vi "Data Receiver_mod.vi"() -> ()   [LabVIEW 2024]
doc: "Demonstrates how to open a connection to a specified host and port, read the data being sent to the port, and display the data on a chart. This VI is designed to stop if the TCP connection is terminated.\n\n<B>Note:</B> Requires the Simple Data Server.vi located in the same library as this VI."
uses:
  <vilib>/Utility/TDMS File Viewer/NI_TDMS File Viewer.lvlib
panel:
  out "Time":string
  out "Bytes to read (dec)":i32
  out "Bytes to read (hex)":string
  out "Complete String after 'Bytes to read'":string
  out "Peak Powers":string[][](array[string])
  out "Peak Wavelengths":string[][](array[string])
  out "System Status":string[][](array[string])
  out "Qty of FBG's":string[](array[string])
  out "OpticalLineNumber":string[](array[string])
  out "Date":string
  out "LineNumber":string
  out "Qty of Optical Lines":string
  in  "Start":bool
  in  "stop":bool
  in  "Address":string="127.0.0.1"
  in  "Port":u16=2055 min=1025 step=1
  # "Instructions:\n1. Adjust the IP address and Port.\n2. Press START."
  # "Separated data"
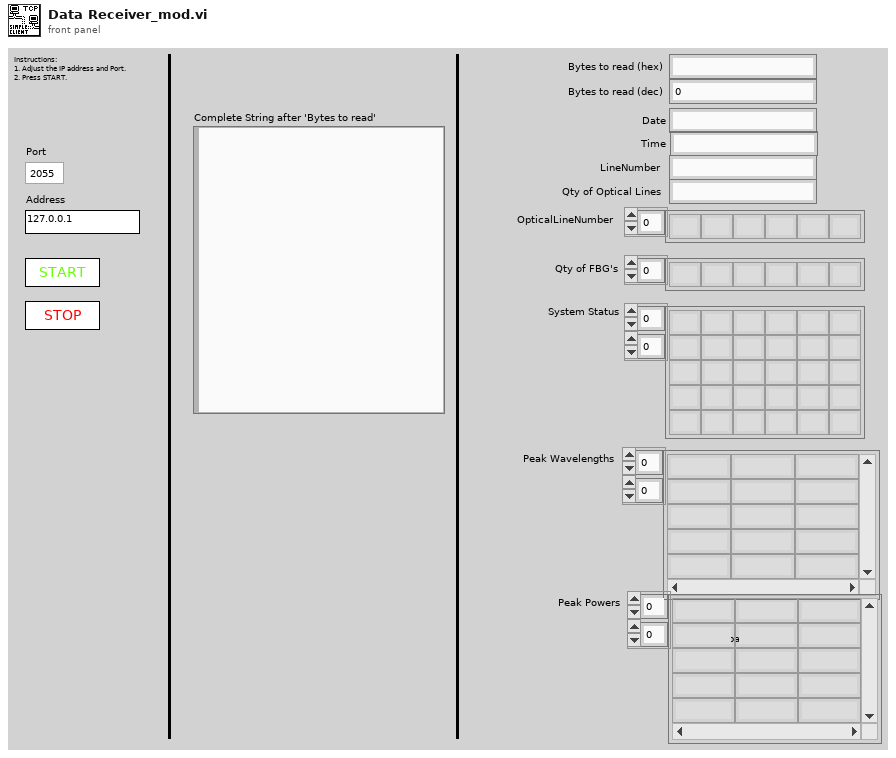
[diagram p1: front panel]
types:
  T1 = enum16{"open", "replace", "create", "open or create", "replace or create", "replace or create with confirmation"}
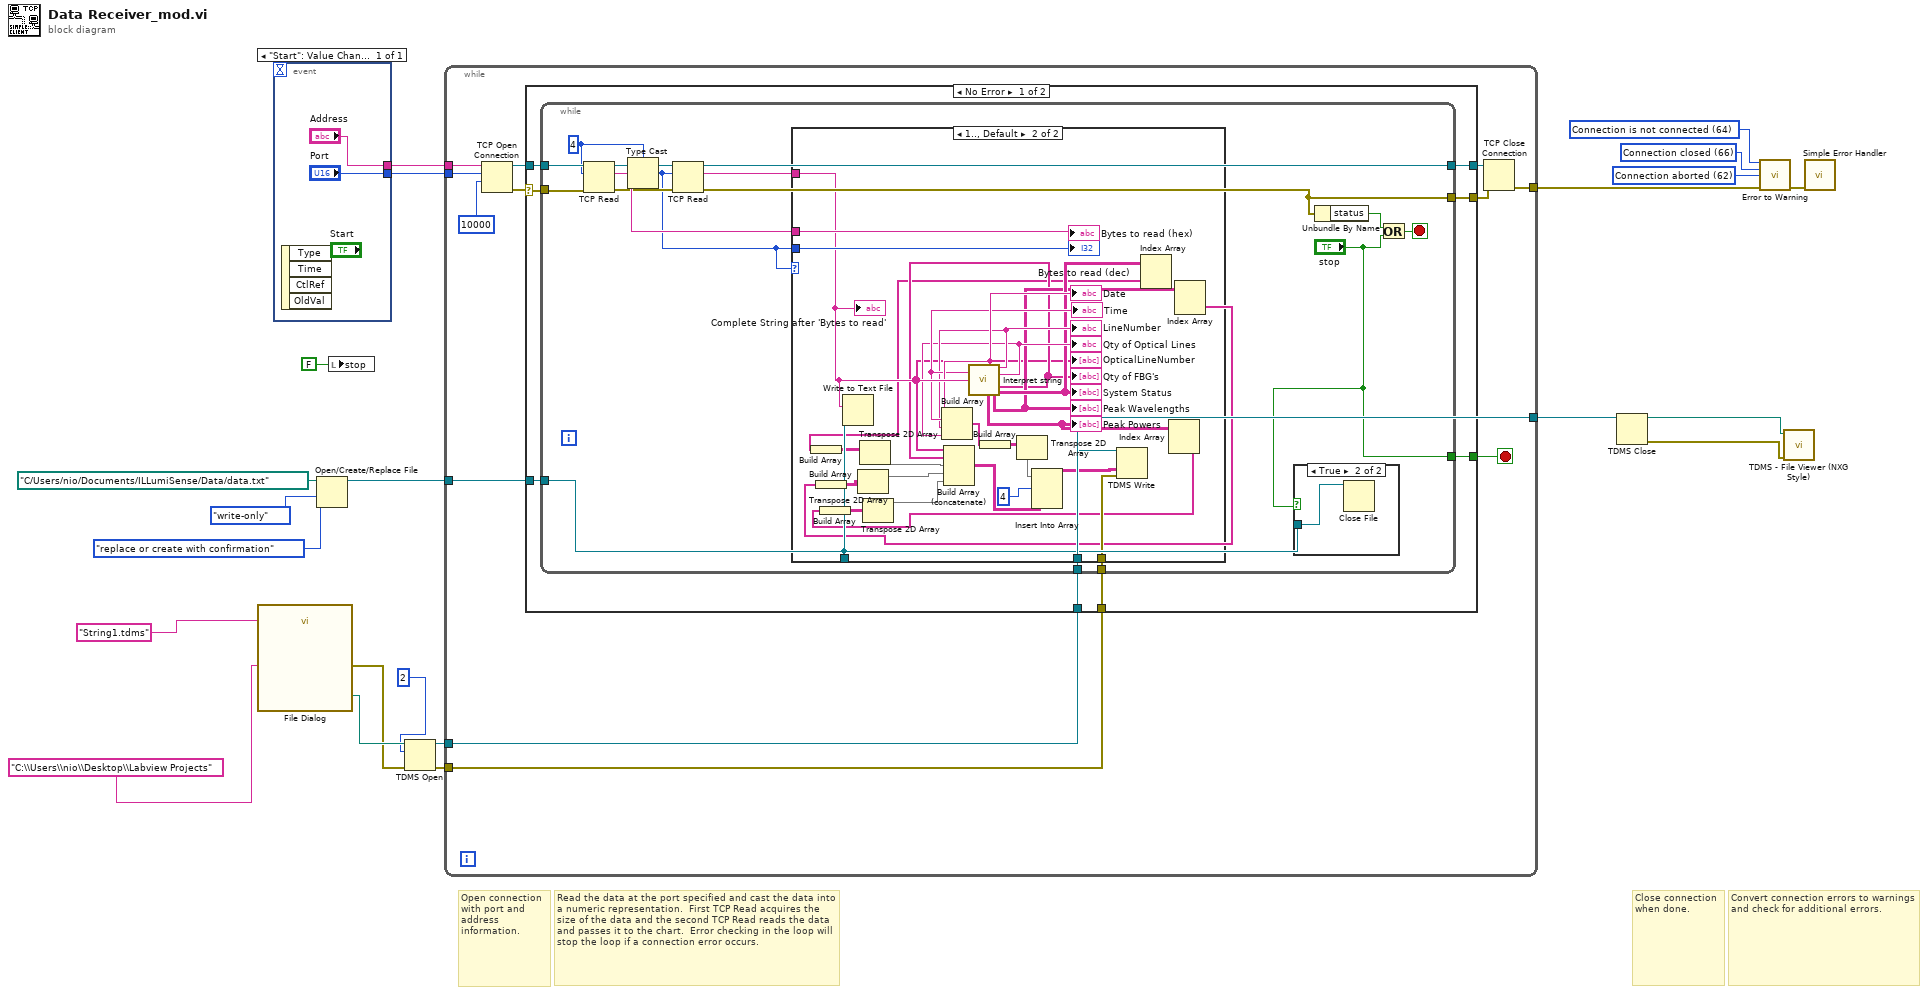
[diagram p0: block diagram]
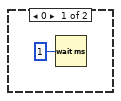
[diagram p3: hidden frame]
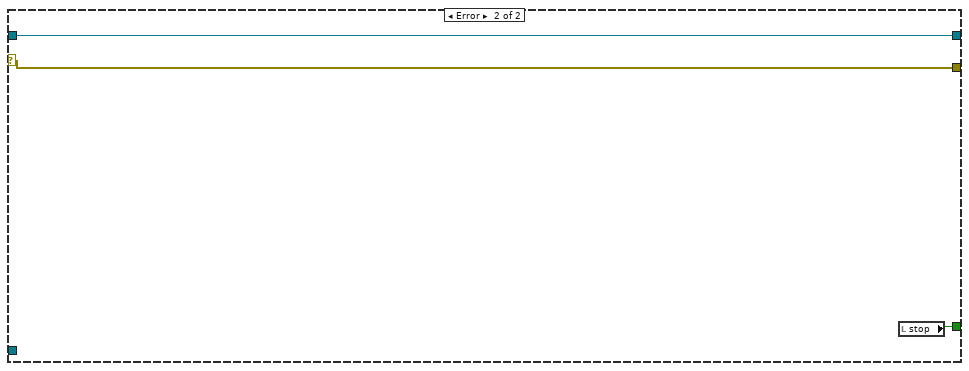
[diagram p4: hidden frame]
diagram:
  w18 = 62 items=["No Error", "Argument Error", "Memory Full", "Out of Zone", "End of File", "File Already Open", "Generic File IO Error", "File Not Found", "File Permission Error", "Disk Full", "Duplicate Path", "Too Many Files Open", "Not Enabled", "Resource File Not Found", "Cannot Add Resource", "Resource Not Found", "Image Not Found", "Image Memory Error", "Pen Does Not Exist", "Config Bad Type", "Config Token Not Found", "Config Parse Error", "Config Memory Error", "Bad External Code Format", "Bad External Code Offset", "External Code Not Present", "Null Window", "Destroy Window Mixup", "Null Menu", "Print Aborted", "Bad Print Record", "Print Driver Error", "Windows Error During Print", "Memory Error During Print", "Print Dialog Error", "Generic Print Error", "Invalid Device Refnum", "Device Not Found", "Device Parameter Error", "Device Unit Error", "Can't Open Device", "Device Call Aborted", "Generic Error", "Cancelled By User", "Object ID Too Low", "Object ID Too High", "Object Not In Heap", "Unknown Heap", "Bad DefProc ID", "DefProc Not In Table", "Message Out Of Range", "Null Method", "Unknown Message", "Manager Call Not Supported", "Bad address", "Connection In progress", "Connection timed out", "Connection is already in progress", "Network attribute not supported", "Network error", "Address in use", "System out of memory", "Connection aborted", "Connection refused", "Connection is not connected", "Connection is already connected", "Connection closed", "Initialize error (interapplication manager)", "Bad occurrence", "Wait on unbound occurrence handler", "Occurrence queue overflow", "Bad path", "Semaphore not signaled", "Unrecognized type (interapplication manager)"] ("1st Error to Convert")
  w19 = 66 items=["No Error", "Argument Error", "Memory Full", "Out of Zone", "End of File", "File Already Open", "Generic File IO Error", "File Not Found", "File Permission Error", "Disk Full", "Duplicate Path", "Too Many Files Open", "Not Enabled", "Resource File Not Found", "Cannot Add Resource", "Resource Not Found", "Image Not Found", "Image Memory Error", "Pen Does Not Exist", "Config Bad Type", "Config Token Not Found", "Config Parse Error", "Config Memory Error", "Bad External Code Format", "Bad External Code Offset", "External Code Not Present", "Null Window", "Destroy Window Mixup", "Null Menu", "Print Aborted", "Bad Print Record", "Print Driver Error", "Windows Error During Print", "Memory Error During Print", "Print Dialog Error", "Generic Print Error", "Invalid Device Refnum", "Device Not Found", "Device Parameter Error", "Device Unit Error", "Can't Open Device", "Device Call Aborted", "Generic Error", "Cancelled By User", "Object ID Too Low", "Object ID Too High", "Object Not In Heap", "Unknown Heap", "Bad DefProc ID", "DefProc Not In Table", "Message Out Of Range", "Null Method", "Unknown Message", "Manager Call Not Supported", "Bad address", "Connection In progress", "Connection timed out", "Connection is already in progress", "Network attribute not supported", "Network error", "Address in use", "System out of memory", "Connection aborted", "Connection refused", "Connection is not connected", "Connection is already connected", "Connection closed", "Initialize error (interapplication manager)", "Bad occurrence", "Wait on unbound occurrence handler", "Occurrence queue overflow", "Bad path", "Semaphore not signaled", "Unrecognized type (interapplication manager)"] ("1st Error to Convert")
  w20 = 64 items=["No Error", "Argument Error", "Memory Full", "Out of Zone", "End of File", "File Already Open", "Generic File IO Error", "File Not Found", "File Permission Error", "Disk Full", "Duplicate Path", "Too Many Files Open", "Not Enabled", "Resource File Not Found", "Cannot Add Resource", "Resource Not Found", "Image Not Found", "Image Memory Error", "Pen Does Not Exist", "Config Bad Type", "Config Token Not Found", "Config Parse Error", "Config Memory Error", "Bad External Code Format", "Bad External Code Offset", "External Code Not Present", "Null Window", "Destroy Window Mixup", "Null Menu", "Print Aborted", "Bad Print Record", "Print Driver Error", "Windows Error During Print", "Memory Error During Print", "Print Dialog Error", "Generic Print Error", "Invalid Device Refnum", "Device Not Found", "Device Parameter Error", "Device Unit Error", "Can't Open Device", "Device Call Aborted", "Generic Error", "Cancelled By User", "Object ID Too Low", "Object ID Too High", "Object Not In Heap", "Unknown Heap", "Bad DefProc ID", "DefProc Not In Table", "Message Out Of Range", "Null Method", "Unknown Message", "Manager Call Not Supported", "Bad address", "Connection In progress", "Connection timed out", "Connection is already in progress", "Network attribute not supported", "Network error", "Address in use", "System out of memory", "Connection aborted", "Connection refused", "Connection is not connected", "Connection is already connected", "Connection closed", "Initialize error (interapplication manager)", "Bad occurrence", "Wait on unbound occurrence handler", "Occurrence queue overflow", "Bad path", "Semaphore not signaled", "Unrecognized type (interapplication manager)"] ("1st Error to Convert")
  # "Convert connection errors to warnings and check for additional errors."
  # "Close connection when done."
  # "Read the data at the port specified and cast the data into a numeric representation.  First TCP Read acquires the size of the data and the second TCP Read reads the data and passes it to the chart.  Error checking in the loop will stop the loop if a connection error occurs."
  # "Open connection\nwith port and \naddress information."
  n1 = call "File Dialog"("prompt"="C:\\Users\\nio\\Desktop\\Labview Projects", "default name"="String1.tdms") -> ("selected path"=w8:path, "error out"=w7:errorcluster)  [unwired: 10 in, 2 out]
  n2 = event shown="[0] \"Start\": Value Change" {
    selector: _ -> [_]
    dyn-events: _ -> [_]
    timeout: _ -> [_]
    tunnel: ["Address"] -> w17
    tunnel: ["Port"] -> w16
    event "Start": Value Change {
      n3 = event-data() -> ()  [unwired: 1 in, 4 out]
    }
  }
  n4 = Open/Create/Replace File(file path (use dialog)=path "C:/Users/nio/Documents/ILLumiSense/Data/data.txt", operation (0:open)=T1."replace or create with confirmation", access (0:read/write)=enum16{"read/write", "read-only", "write-only"}."write-only") -> (refnum out=w11:refnum<file>)  [unwired: 3 in, 2 out]
  n5 = local write "stop"(FALSE ("stop")) -> ()
  n6 = TDMS Open(8:w7, 10:u32 2 ("milliseconds to wait"), 11:w8) -> (0:w4:errorcluster, 3:w5:refnum<k34>)  [unwired: 4 in]
  n7 = while {
    tunnel: [w33] -> w22
    tunnel: w17 -> [w32]
    tunnel: w16 -> [w31]
    tunnel: w11 -> [w28]
    tunnel: w5 -> [w25]
    tunnel: w4 -> [w26]
    tunnel: [w25] -> w3
    stop <- w30 stop-if-true
    n8 = TCP Open Connection(address=w32, remote port or service name=w31, timeout ms (60000)=10000) -> (connection ID=w34:refnum<k5>, error out=w29:errorcluster)  [unwired: 2 in]
    n9 = case shown="No Error" w29 {
      selector: w29 -> [w40 w94]
      tunnel: [w44 w94] -> w36
      tunnel: [w43 w95] -> w35
      tunnel: w34 -> [w42 w95]
      tunnel: [w41 w93] -> w30
      tunnel: w28 -> [w39 _]
      tunnel: w25 -> [w38 _]
      tunnel: w26 -> [w37 _]
      frame No Error {
        n10 = while {
          tunnel: w40 -> [w57]
          tunnel: w42 -> [w58]
          tunnel: [w59] -> w43
          tunnel: [w56] -> w44
          tunnel: ["stop"] -> w41
          tunnel: w39 -> [w49]
          tunnel: w38 -> [w46]
          tunnel: w37 -> [w45]
          stop <- w54 stop-if-true
          w48 = 4
          n11 = TCP Read(connection ID=w58, bytes to read=w48, error in (no error)=w57) -> (connection ID out=w60:refnum<k5>, data out=w53:string, error out=w51:errorcluster)  [unwired: 2 in]
          n12 = Type Cast(type=w48, x=w53) -> (*(type *) &x=w47:i32)
          n13 = TCP Read(connection ID=w60, bytes to read=w47, error in (no error)=w51) -> (connection ID out=w59:refnum<k5>, data out=w52:string, error out=w56:errorcluster)  [unwired: 2 in]
          n14 = case shown="1.., Default" w47 {
            tunnel: w53 -> [_ w92]
            tunnel: w52 -> [_ w89]
            tunnel: w47 -> [_ w91]
            tunnel: w49 -> [_ w90]
            tunnel: w46 -> [_ w88]
            tunnel: w45 -> [_ w87]
            frame 0 {
              n15 = Wait (ms)(milliseconds to wait=u32 1) -> ()  [unwired: 1 out]
            }
            frame 1.., Default {
              n16 = Write to Text File(file (use dialog)=w90, text=w89) -> ()  [unwired: 2 in, 3 out]
              n17 = call "Interpret string.vi"("Spreadsheet string"=w89) -> ("Time"=w85:string, "Date"=w86:string, "LineNumber"=w84:string, "Qty of Optical Lines"=w83:string, "OpticalLineNumber"=w78:string[], "Qty of FBG's"=w79:string[], "Peak Powers"=w80:string[][], "Peak Wavelengths"=w81:string[][], "System Status"=w82:string[][])  [unwired: 6 in]
              "Qty of Optical Lines" <- w83
              "LineNumber" <- w84
              "Date" <- w86
              "OpticalLineNumber" <- w78
              "Qty of FBG's" <- w79
              "System Status" <- w82
              "Peak Wavelengths" <- w81
              "Peak Powers" <- w80
              "Time" <- w85
              n18 = Build Array(w86, w85, w84, w83) -> (w68:string[])
              n19 = Build Array(w68) -> (w67:string[][])
              n20 = Transpose 2D Array(2D array=w67) -> (transposed array=w66:string[][])
              n21 = Index Array(array=w82) -> (element=w77:string[])  [unwired: 2 in]
              n22 = Build Array(w77) -> (w76:string[][])
              n23 = Transpose 2D Array(2D array=w76) -> (transposed array=w75:string[][])
              n24 = Index Array(array=w80) -> (element=w71:string[])  [unwired: 2 in]
              n25 = Build Array(w71) -> (w70:string[][])
              n26 = Transpose 2D Array(2D array=w70) -> (transposed array=w69:string[][])
              n27 = Index Array(array=w81) -> (element=w73:string[])  [unwired: 2 in]
              n28 = Build Array(w73) -> (w74:string[][])
              n29 = Transpose 2D Array(2D array=w74) -> (transposed array=w72:string[][])
              n30 = Build Array (concatenate)(w78, w79, w75, w72, w69) -> (w65:string[][])
              n31 = Insert Into Array(array=w66, index (row)=4 ("disabled index (col)"), new element=w65) -> (w64:string[][])  [unwired: 1 in]
              n32 = TDMS Write(0:w88, 9:w64, 11:w87) -> ()  [unwired: 3 in, 4 out]
              "Complete String after 'Bytes to read'" <- w89
              "Bytes to read (hex)" <- w92
              "Bytes to read (dec)" <- w91
            }
          }
          n33 = case shown="True" "stop" {
            tunnel: w49 -> [_ w61]
            frame False {
            }
            frame True {
              n34 = Close File(refnum=w61) -> ()  [unwired: 1 in, 2 out]
            }
          }
          n35 = Unbundle By Name(w56) -> ("status"=w55:bool)
          n36 = Or(x=w55, y="stop") -> (x .or. y?=w54:bool)
        }
      }
      frame Error {
        n37 = local read "stop"() -> (w93:bool)
      }
    }
    n38 = TCP Close Connection(connection ID=w35, error in (no error)=w36) -> (error out=w33:errorcluster)  [unwired: 1 in, 1 out]
  }
  n39 = TDMS Close(11:w3) -> (0:w1:errorcluster, 3:w2:path)  [unwired: 1 in]
  n40 = call <vilib>:"Error to Warning.vi"("1st Error to Convert"=w20, "2nd Error to Convert"=w19, "3rd Error to Convert"=w18, "error in"=w22) -> ("warning out"=w21:errorcluster)  [unwired: 11 in]
  n41 = call <vilib>:"TDMS - File Viewer (NXG Style).vi"("error in"=w1, "file in"=w2) -> ()  [unwired: 8 in, 2 out]
  n42 = call <vilib>:"Simple Error Handler.vi"("error in (no error)"=w21) -> ()  [unwired: 4 in, 5 out]
